vi "piezoWriteOpen.vi"() -> ()   [LabVIEW 2017]
uses:
  <vilib>/DAQmx/write.llb/DAQmx Write (Analog 1D DBL 1Chan NSamp).vi
  <vilib>/DAQmx/write.llb/DAQmx Write (Analog DBL 1Chan 1Samp).vi
  globalDevices.vi
  <vilib>/DAQmx/create/channels.llb/DAQmx Create Channel (AO-Voltage-Basic).vi
  <vilib>/DAQmx/configure/timing.llb/DAQmx Timing (Sample Clock).vi
  <vilib>/DAQmx/miscellaneous.llb/DAQmx Fill In Error Info.vi
panel:
  out "Waveform Graph":dbl[](graph)
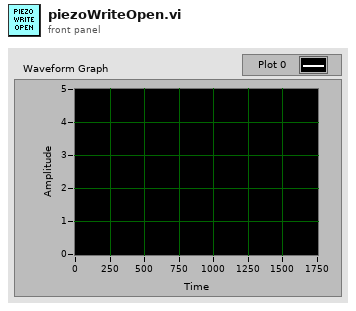
[diagram p1: front panel]
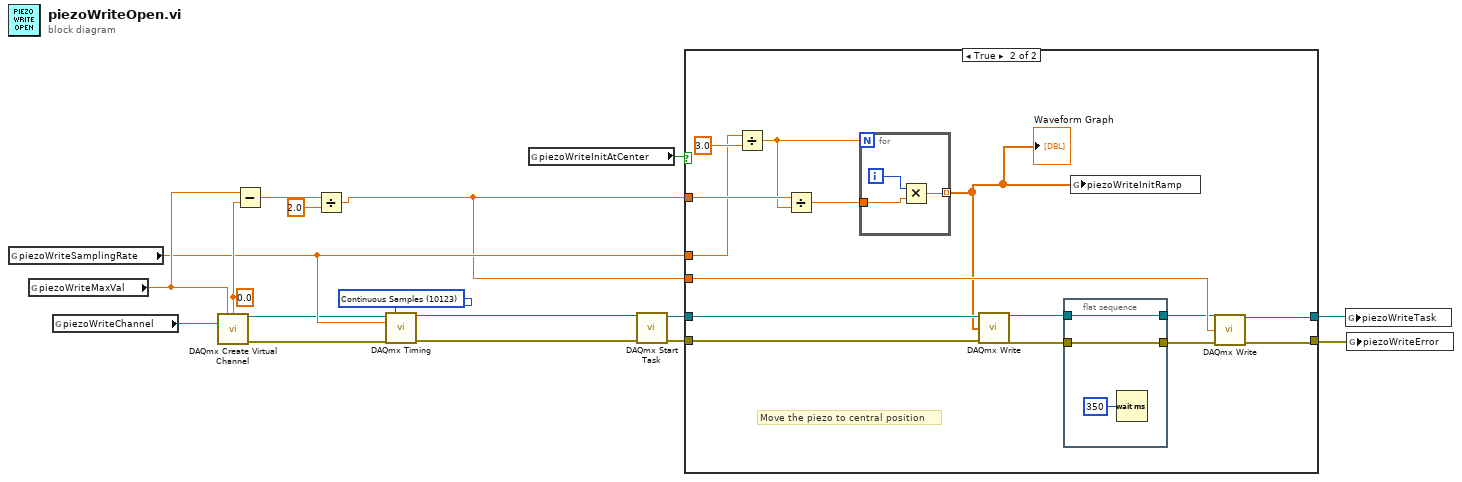
[diagram p0: block diagram]
diagram:
  w10 = 10123 items=["Finite Samples"=10178, "Continuous Samples"=10123, "Hardware Timed Single Point"=12522] ("sample mode")
  w15 = 0.0 ("minimum value")
  n1 = global read "globalDevices.vi" "piezoWriteSamplingRate"() -> (w13:dbl)
  n2 = global read "globalDevices.vi" "piezoWriteMaxVal"() -> (w16:dbl)
  n3 = global read "globalDevices.vi" "piezoWriteChannel"() -> (w17:tag)
  n4 = call-poly <vilib>:"DAQmx Create Virtual Channel.vi"("maximum value"=w16, "minimum value"=w15, "physical channels"=w17) -> ("task out"=w9:refnum<k21>, "error out"=w8:errorcluster)  [unwired: 11 in]
  n5 = Subtract(x=w16, y=w15) -> (x-y=w14:dbl)
  n6 = Divide(x=w14, y=2.0) -> (x/y=w6:dbl)
  n7 = call-poly <vilib>:"DAQmx Timing.vi"("task/channels in"=w9, "sample mode"=w10, "rate"=w13, "error in"=w8) -> ("task out"=w5:refnum<k21>, "error out"=w4:errorcluster)  [unwired: 10 in]
  n8 = global read "globalDevices.vi" "piezoWriteInitAtCenter"() -> (w1:bool)
  n9 = call <vilib>:"DAQmx Start Task.vi"("task/channels in"=w5, "error in"=w4) -> ("task out"=w2:refnum<k21>, "error out"=w3:errorcluster)  [unwired: 12 in]
  n10 = case shown="True" w1 {
    tunnel: w2 -> [w19 w28]
    tunnel: w3 -> [w18 w29]
    tunnel: w6 -> [_ w33]
    tunnel: w13 -> [_ w30]
    tunnel: [w19 w27] -> w12
    tunnel: [w18 w26] -> w11
    tunnel: w6 -> [_ w25]
    frame False {
    }
    frame True {
      # "Move the piezo to central position"
      n11 = Divide(x=w30, y=3.0) -> (x/y=w32:dbl)
      n12 = Divide(x=w33, y=w32) -> (x/y=w31:dbl)
      n13 = for {
        N: w32 -> [_]
        tunnel: w31 -> [w39]
        tunnel: [w38] -> w20 mode=indexing
        i -> [w40]
        n14 = Multiply(x=w40, y=w39) -> (x*y=w38:dbl)
      }
      "Waveform Graph" <- w20
      n15 = call-poly <vilib>:"DAQmx Write.vi"("task/channels in"=w28, "data"=w20, "error in"=w29) -> ("task out"=w24:refnum<k21>, "error out"=w21:errorcluster)  [unwired: 10 in, 1 out]
      n16 = flat-sequence {
        tunnel: w24 -> [w37]
        tunnel: [w37] -> w23
        tunnel: [w36] -> w22
        tunnel: w21 -> [w36]
        frame #0 {
          n17 = Wait (ms)(milliseconds to wait=u32 350) -> ()  [unwired: 1 out]
        }
      }
      n18 = global write "globalDevices.vi" "piezoWriteInitRamp"(w20) -> ()
      n19 = call-poly <vilib>:"DAQmx Write.vi"("task/channels in"=w23, "data"=w25, "error in"=w22) -> ("task out"=w27:refnum<k21>, "error out"=w26:errorcluster)  [unwired: 10 in, 1 out]
    }
  }
  n20 = global write "globalDevices.vi" "piezoWriteTask"(w12) -> ()
  n21 = global write "globalDevices.vi" "piezoWriteError"(w11) -> ()
